vi "Robot Global Data.vi"() -> ()   [LabVIEW 2015]
doc: "This global VI can contain as many global variables as you need. Place a control on the panel, give it a good name. To read or write to it from a VI, drag the icon to the diagram of that VI. You can also drag from the project. Click on the node to change which global you access. You shouldn't have multiple locations writing to a global or it will cause a race-condition."
uses:
  <vilib>/Rock Robotics/WPI/Camera/WPI_CameraImageSize.ctl
  <vilib>/Rock Robotics/WPI/DriverStation/WPI_DriverStationRobotMode2.ctl
panel:
  in  "CamTargetMem":dbl=-0.026
  in  "CamTargetReal":dbl=-0.026
  out "LR":bool=TRUE
  in  "Slew":dbl=0.2
  in  "Pins / Intake timing":dbl=550.0
  out "tapesModArm":bool
  out "Camera Target":dbl=-0.026
  in  "arm slow spot normal":dbl=0.1
  in  "arm slow spot cdf":dbl=0.05
  out "1-slider":bool
  in  "camera switch":bool=TRUE
  in  "arm speed shovel":dbl=0.45
  in  "arm speed normal":dbl=0.33
  out "finishedRtweak":bool
  out "finishedLtweak":bool
  in  "Starting Position":i32=3
  in  "Defense to Cross":i32=6
  out "4?":bool
  out "1-Button 8":bool
  out "1-Button 5":bool
  out "arm pot unfiltered":dbl=0.9048439735036312
  in  "Heading":dbl=298.75
  in  "Pitch":dbl=1.83
  in  "Yaw":dbl=-61.24
  in  "IsPracticeBot?":bool=TRUE
  in  "IR dist to CDF":dbl=0.021972654
  in  "left num":i8
  in  "climb num":i32
  in  "right num":i8
  in  "arm speed slow":dbl=0.1
  in  "arm slow spot":dbl=0.1
  in  "Left 2":bool
  in  "Right 2":bool
  in  "arm out":dbl=-0.0
  in  "arm speed":dbl=0.33
  in  "ball dist thresh":dbl=1.8
  in  "IR dist to ball":dbl=0.09887694300000001
  out "retainer override":bool
  in  "retainer num":i16=2
  in  "in ctl num":i16
  out "in pos override":bool
  in  "arm override":bool
  in  "arm stow":dbl=0.76
  in  "arm extended":dbl=0.32
  in  "climb":bool
  out "PTO speed":dbl
  in  "Shoot!":bool
  in  "In ctl 2":bool=TRUE
  in  "In ctl 1":bool
  in  "In pos":bool
  in  "Retainer 2":bool=TRUE
  in  "Retainer":bool=TRUE
  in  "Right":bool
  in  "Left":bool
  in  "climb 2":bool
  out "center Y":dbl
  out "center X":dbl
  out "Distance (cam)":dbl
  in  "Shot Selector":bool
  out "arm pot":dbl=0.9047725592758695
  in  "Arm Control":dbl(knob)=1.0 scale=-1.0..1.0
  out "shift state":bool=TRUE
  in  "PTO Engaged":bool
  out "Shift Lockout?":bool
  out "Distance (enc.)":dbl=-438.38479125
  out "Velocity":dbl
  out "1-Trigger":bool
  out "1-TopRight":bool
  out "1-TopLeft":bool
  out "1-Zrotate":dbl
  out "1-X":dbl
  out "1-Y":dbl
  out "1-TopCenter":bool
  in  "Robot Mode":T1=enum."Teleop Disabled"
  in  "image size":T2=enum."320x240"
  in  "Enable Vision":bool
  # "Once these are true, tapes are in \"tweak mode\""
  # "Arm-related settings"
  # "After tapes go up arms are locked in stow"
  # "Soft limits"
  # "Speed (2 stage bang bang)"
  # "Dist to start slow. Changes during auto-cdf to hit harder. Leftmost one is one used by code"
  # "Same idea. More power on cdf"
  # "Desired arm power"
  # "Tape Measures"
  # "potentiometer readings"
  # "CHANGE MEM"
  # "SENSOR READINGS"
  # "2BALL = MEM - .01"
  # "MEM = CameraTarget3 (PT)"
  # "00        - normal\n01 10   - PTO engaged\n11        - climb"
  # "00        - out\n01 10   - off\n11        - in"
  # "This reads a jumper to set arms according\nto comp or practice bot. Lifesaver in build\nseason after we wrecked an arm assembly"
  # "00        - off\n01 10   - on\n11        - auto"
  # "In order to not\ncrash catapult\nwith retainer pins\nor intake:"
  # "Close"
  # "Down"
  # "Up"
  # "Far"
  # "Simulation of the button box that we use to guide our building\nof the box. Makes it easier to virtually manipulate controls if its identical\nto our physical control scheme"
  # "auto selectors"
  # "Joystick controls go here"
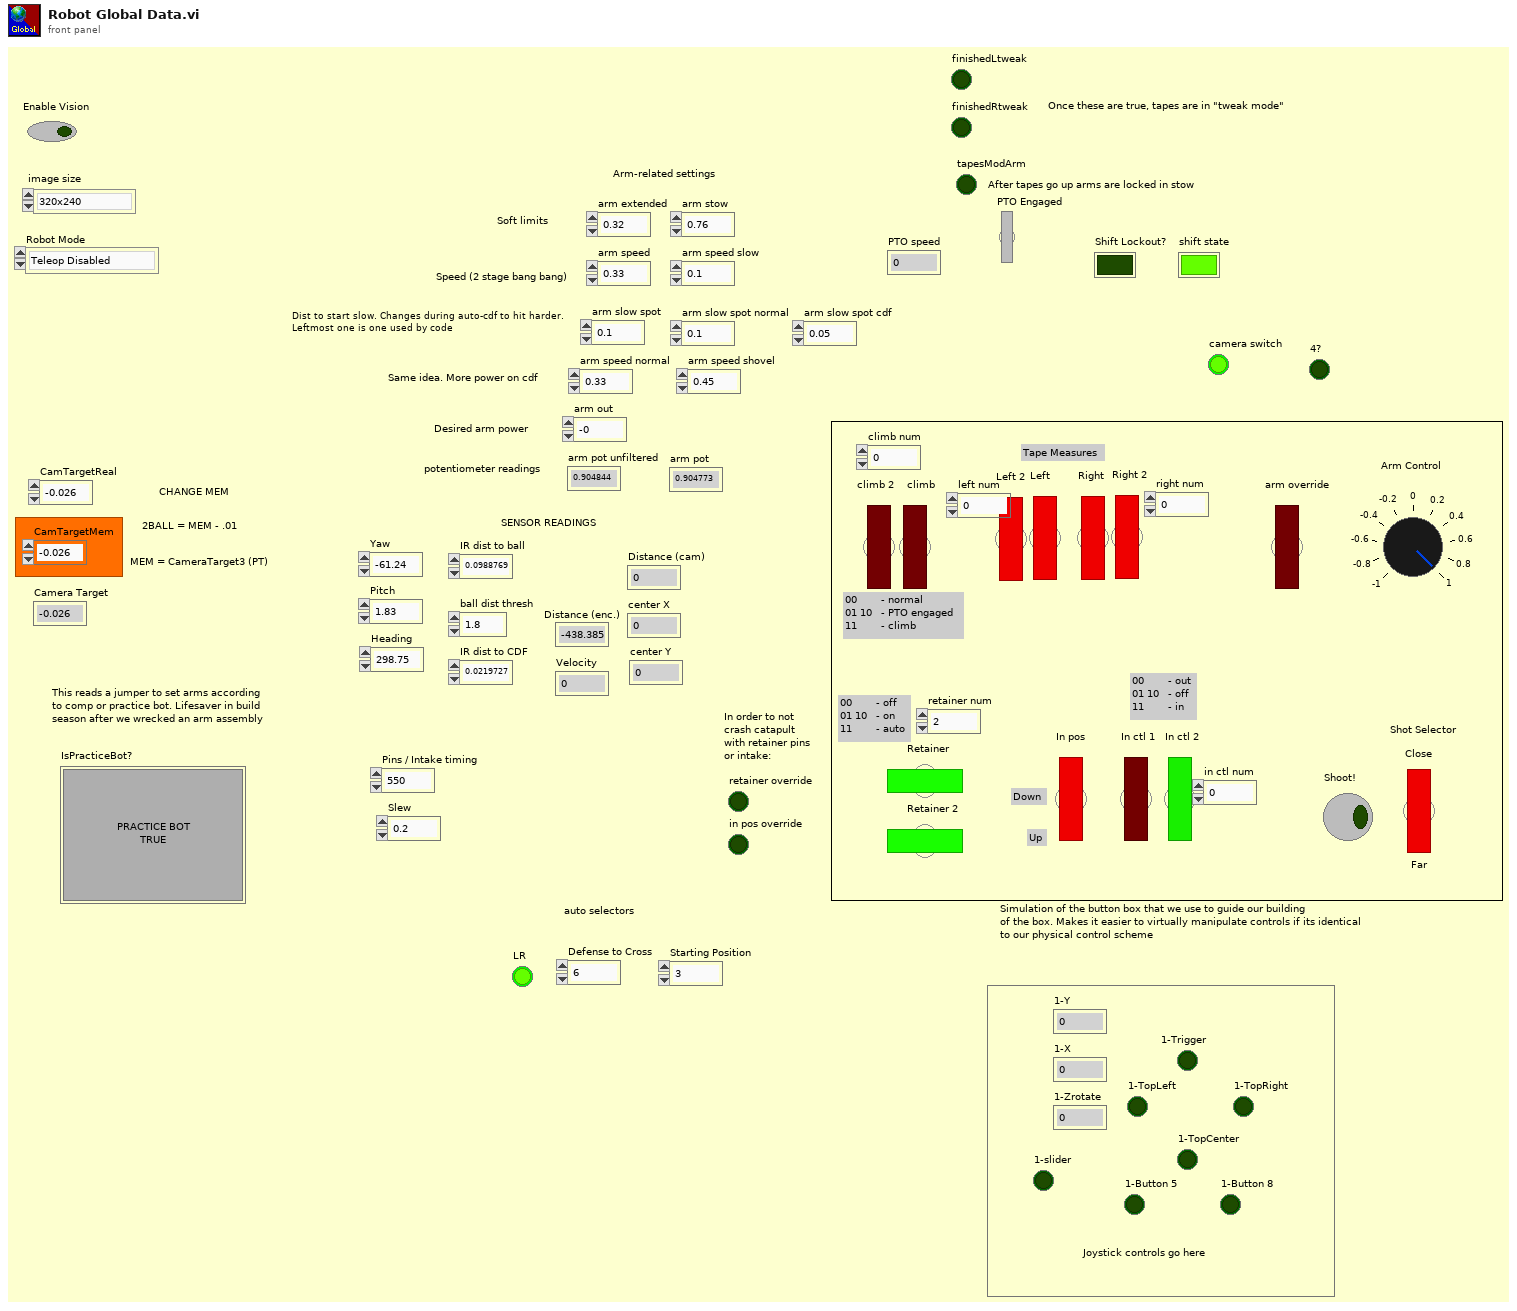
[diagram p1: front panel]
types:
  T1 = typedef "WPI_DriverStationRobotMode2.ctl" = enum16{"Autonomous Disabled", "Autonomous Enabled", "Teleop Disabled", "Teleop Enabled", "Disconnected", "Finish", "Test Disabled", "Test Enabled", "Emergency Stopped"}
  T2 = typedef "WPI_CameraImageSize.ctl" = enum16{"640x480", "320x240", "160x120", "Custom"}
diagram:
